vi "check in tracking state.vi"(6 "tick count":u32, 9 "check in state":bool=TRUE, 11 "state to check in":T1={"x state"={"pos estimate"=0.0, "v estimate"=0.0, "weighted position error sum"=0.0, "photon count"=0, "transmit tick count"=0, "axis number"=0, "px (levels^2)"=0.0, "pxv (levels^2/ticks)"=0.0, "pv (levels^2/ticks^2)"=0.0, "vel diff (levels^2/ticks^3)"=0.0, "gx"=0.0, "rtwiddle"=0.0, "photon count ch0"=0, "photon count ch1"=0, "Dx -levels^2/ticks"=0.0}, "y state"={"pos estimate"=0.0, "v estimate"=0.0, "weighted position error sum"=0.0, "photon count"=0, "transmit tick count"=0, "axis number"=1, "px (levels^2)"=0.0, "pxv (levels^2/ticks)"=0.0, "pv (levels^2/ticks^2)"=0.0, "vel diff (levels^2/ticks^3)"=0.0, "gx"=0.0, "rtwiddle"=0.0, "photon count ch0"=0, "photon count ch1"=0, "Dx -levels^2/ticks"=0.0}, "z state"={"pos estimate"=0.0, "v estimate"=0.0, "weighted position error sum"=0.0, "photon count"=0, "transmit tick count"=0, "axis number"=2, "px (levels^2)"=0.0, "pxv (levels^2/ticks)"=0.0, "pv (levels^2/ticks^2)"=0.0, "vel diff (levels^2/ticks^3)"=0.0, "gx"=0.0, "rtwiddle"=0.0, "photon count ch0"=0, "photon count ch1"=0, "Dx -levels^2/ticks"=0.0}, "spot number"=0}) -> ()   [LabVIEW 2010]
uses:
  kalman 3-axis state.ctl
  integrating single axis kalman state.ctl
  <vilib>/rvi/DataTransferAndStorage/Container/XNode/niFpgaContainer.xnode
  <vilib>/rvi/Memory/Memory_Emulation/nirvimemoryEmulationManagerCache_GetValue.vi
  <vilib>/rvi/DataTransferAndStorage/Container/Common/niFpgaContainerGetUniqueNameForEmu.vi
  <vilib>/rvi/Memory/Memory_Emulation/nirvimemoryEmulationManagerCache_InsertValue.vi
  <vilib>/Utility/error.llb/Clear Errors.vi
  <vilib>/rvi/Memory/Memory_Emulation/nirvimemoryEmulationManagerCache_SetValue.vi
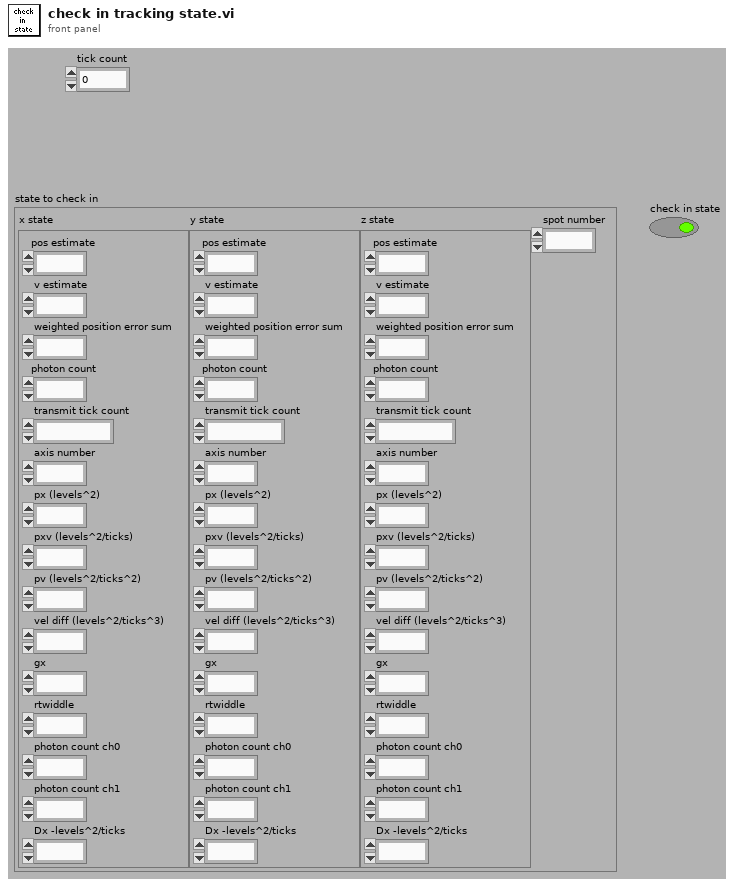
[diagram p1: front panel]
types:
  T1 = typedef "kalman 3-axis state.ctl" = cluster{"x state":T2, "y state":T2, "z state":T2, "spot number":u8}
  T2 = typedef "integrating single axis kalman state.ctl" = cluster{"pos estimate":fxp<+/-,32,16>, "v estimate":fxp<+/-,16,0>, "weighted position error sum":fxp<+/-,32,32>, "photon count":u32, "transmit tick count":u32, "axis number":u8, "px (levels^2)":fxp<+,32,19>, "pxv (levels^2/ticks)":fxp<+,32,2>, "pv (levels^2/ticks^2)":fxp<+,32,-14>, "vel diff (levels^2/ticks^3)":fxp<+,24,-22>, "gx":fxp<+,16,8>, "rtwiddle":fxp<+,16,26>, "photon count ch0":u32, "photon count ch1":u32, "Dx -levels^2/ticks":fxp<+,32,19>}
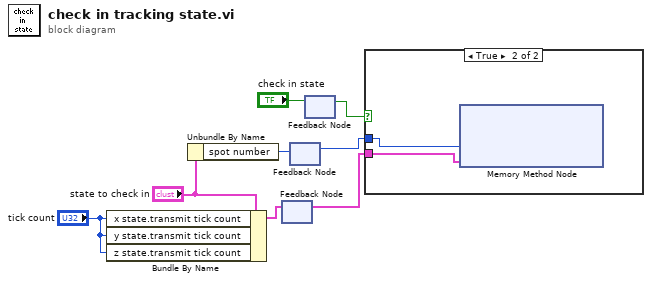
[diagram p0: block diagram]
diagram:
  n1 = Bundle By Name(cluster="state to check in", "x state.transmit tick count"="tick count", "y state.transmit tick count"="tick count", "z state.transmit tick count"="tick count") -> (w2:T1)
  n2 = Unbundle By Name("state to check in") -> ("spot number"=w3:u8)
  n3 = feedback-in #1(w2) -> ()
  n4 = feedback #1() -> (w5:T1)  [unwired: 1 in]
  n5 = feedback-in #2(w3) -> ()
  n6 = feedback #2() -> (w6:u8)  [unwired: 1 in]
  n7 = feedback-in #3("check in state") -> ()
  n8 = feedback #3() -> (w7:bool)  [unwired: 1 in]
  n9 = case shown="True" w7 {
    tunnel: w6 -> [_ w10]
    tunnel: w5 -> [_ w9]
    frame False {
    }
    frame True {
      n10 = xnode ("Memory Method Node")("Address"=w10, "Data"=w9) -> ()  [unwired: 1 in, 1 out]
    }
  }
